vi "Position Data Updated.vi"(8 "error in":errorcluster, 9 "Data":variant, 10 "Point Ident":string, 11 "ITask Actor in":refnum<class "ITask Actor.lvclass">) -> (0 "error out":errorcluster, 3 "ITask Actor out":refnum<class "ITask Actor.lvclass">)   [LabVIEW 2023, in "HAL GOOP4.lvlib" / "ITask Actor.lvlib" / "ITask Actor.lvclass"]
uses:
  ITask Actor.lvclass
  <vilib>/Utility/error.llb/Error Cluster From Error Code.vi
  <vilib>/ErrorRing/Error Ring.xnode
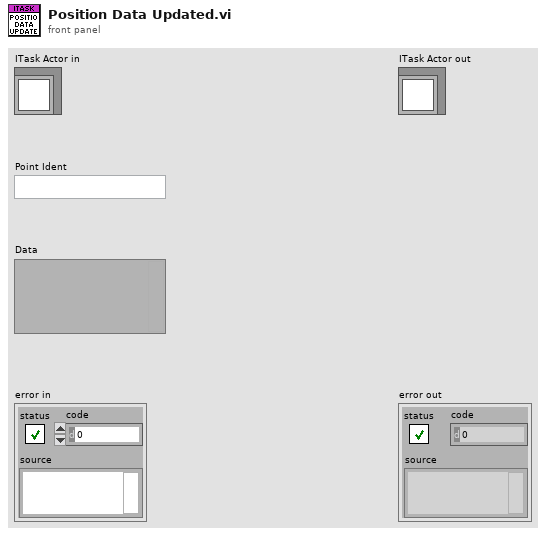
[diagram p1: front panel]
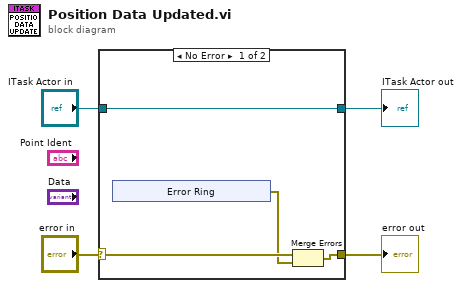
[diagram p0: block diagram]
diagram:
  n1 = case shown="No Error" "error in" {
    selector: "error in" -> [w7 w15]
    tunnel: [w6 w15] -> w3
    tunnel: [w8 w14] -> w1
    tunnel: "ITask Actor in" -> [w8 w14]
    frame No Error {
      n2 = xnode "Error Ring"() -> ("error out"=w5:errorcluster)
      n3 = Merge Errors(w7, w5) -> (w6:errorcluster)
    }
    frame Error {
    }
  }
  "error out" <- w3
  "ITask Actor out" <- w1
